vi "Get SMO Port.vi"(8 "error in (no error)":errorcluster, 11 "Inst.TSL210Instrument in":refnum<class "Inst.TSL210.lvclass">) -> (0 "error out":errorcluster, 2 "Port":u16, 3 "Inst.TSL210Instrument out":refnum<class "Inst.TSL210.lvclass">)   [LabVIEW 2019, in "Inst.TSL210.lvclass"]
uses:
  Inst.TSL210.lvclass
  <userlib>/LevyLab/Instrument Framework/Instrument Types/VSource/Instrument.VSource.lvclass
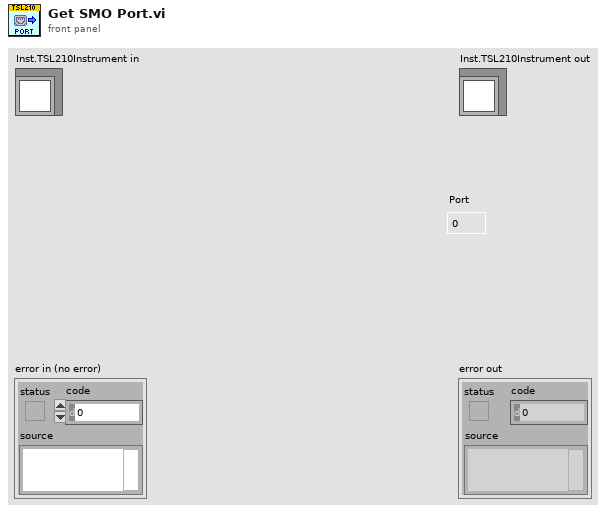
[diagram p1: front panel]
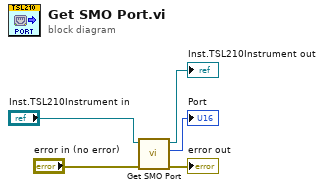
[diagram p0: block diagram]
diagram:
  n1 = call-parent "Get SMO Port.vi"("error in (no error)"="error in (no error)", "Instrument in"="Inst.TSL210Instrument in") -> ("error out"=→"error out":errorcluster, "Port"=→"Port":u16, "Instrument out"=→"Inst.TSL210Instrument out":refnum<class "Inst.TSL210.lvclass">)  [unwired: 7 in]
